vi "uActor_Launch.vi"(6 "Show FP (F)":bool, 8 "error in (no error)":errorcluster, 10 "Actor to Launch":refnum<class "uActor.lvclass">, 11 "Caller Actor in":refnum<class "uActor.lvclass">) -> (0 "error out":errorcluster, 2 "uTransport_uActor":refnum<class "uTransport_uActor.lvclass">, 3 "Caller Actor out":refnum<class "uActor.lvclass">)   [LabVIEW 2021, in "uFramework.lvlib" / "uActor.lvclass"]
doc: "Launch a new Actor. This will be a root actor if no caller actors are wired in."
uses:
  uActor.lvclass
  uTransport_uActor/uTransport_uActor.lvclass
  uTransport_uActor/uTransport_uActor.lvclass/uTransport_uActor.ctl
  uActor.lvclass/uActor.ctl
  uActor.vi
  uMsg/uMsg.lvclass
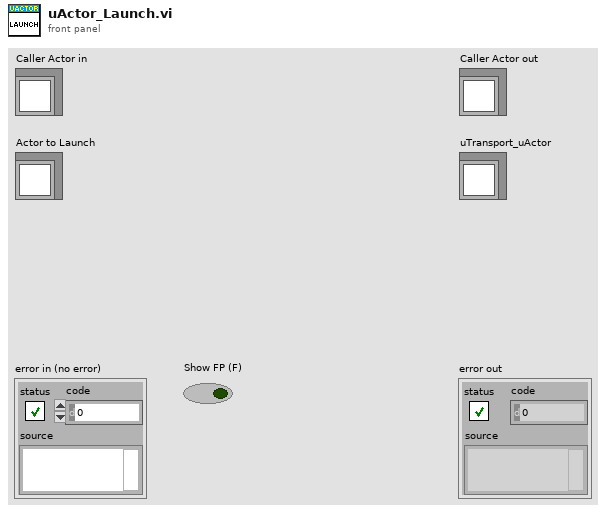
[diagram p1: front panel]
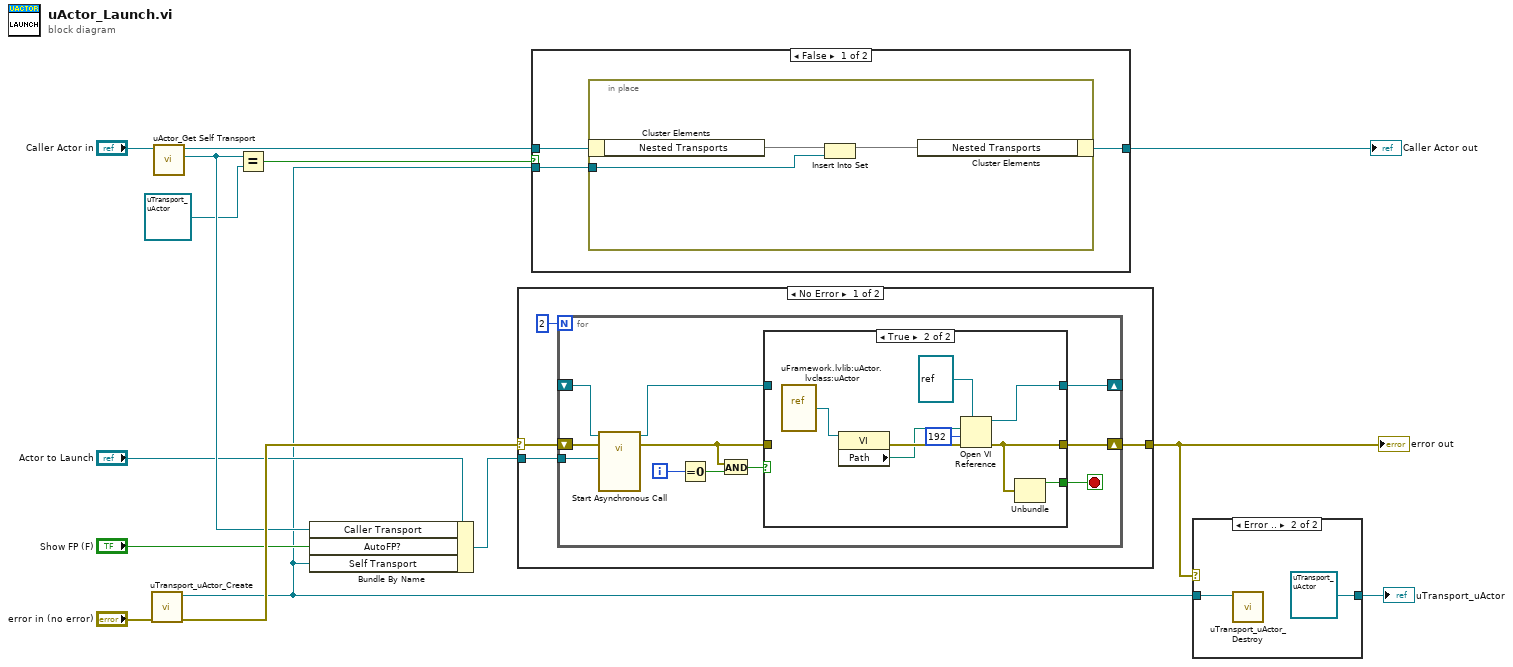
[diagram p0: block diagram]
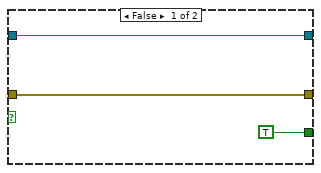
[diagram p2: hidden frame]
diagram:
  n1 = call "uTransport_uActor_Create.vi"("error in (no error)"="error in (no error)") -> ("error out"=w14:errorcluster, "uTransport_uActor out"=w2:refnum<class "uTransport_uActor.lvclass">)  [unwired: 9 in]
  n2 = call "uActor_Get Self Transport.vi"("uActor in"="Caller Actor in") -> ("Actor Transport"=w9:refnum<class "uTransport_uActor.lvclass">, "uActor out"=w7:refnum<class "uActor.lvclass">)  [unwired: 9 in]
  n3 = Equal?(x=w9, y=refnum<class "uTransport_uActor.lvclass"> refnum ("uFramework.lvlib:uTransport_uActor.lvclass")) -> (x = y?=w8:bool)
  n4 = Bundle By Name(cluster="Actor to Launch", "Caller Transport"=w9, "AutoFP?"="Show FP (F)", "Self Transport"=w2) -> (w13:refnum<class "uActor.lvclass">)
  n5 = case shown="No Error" w14 {
    selector: w14 -> [w15 w41]
    tunnel: w13 -> [w18 _]
    tunnel: [w17 w41] -> w5
    frame No Error {
      n6 = for {
        N: 2 -> [_]
        tunnel: w18 -> [w29]
        shift-right: [w25] -> w17
        shift-left: w15 -> [w28]
        shift-right: [w26] -> _
        shift-left: _ -> [w27]
        i -> [w24]
        stop <- w19 stop-if-true
        n7 = call-by-ref "Start Asynchronous Call"(reference=w27, error in=w28, "uActor in"=w29) -> (reference out=w23:refnum<vi>, error out=w20:errorcluster)  [unwired: 9 in, 2 out]
        n8 = Equal To 0?(x=w24) -> (x = 0?=w21:bool)
        n9 = And(x=w20, y=w21) -> (x .and. y?=w22:bool)
        n10 = case shown="True" w22 {
          tunnel: w20 -> [w31 _]
          tunnel: [w32 w35] -> w26
          tunnel: [w31 w34] -> w25
          tunnel: w23 -> [w32 _]
          tunnel: [TRUE w33] -> w19
          frame False {
          }
          frame True {
            n11 = vi-ref "uFramework.lvlib:uActor.lvclass:uActor.vi"() -> (w37:refnum<vi>)
            n12 = property class="VI"(reference=w37) -> (error out=w40:errorcluster, "Path"=w39:path)  [unwired: 1 in, 1 out]
            n13 = Open VI Reference(type specifier VI Refnum (for type only)=refnum<vi> refnum, vi path=w39, options=192, error in (no error)=w40) -> (vi reference=w35:refnum<vi>, error out=w34:errorcluster)  [unwired: 2 in]
            n14 = Unbundle(w34) -> ("status"=w33:bool)  [unwired: 2 out]
          }
        }
      }
    }
    frame Error {
    }
  }
  "error out" <- w5
  n15 = case shown="False" w8 {
    tunnel: w7 -> [w44 w48]
    tunnel: [w42 w48] -> w6
    tunnel: w2 -> [w43 _]
    frame False {
      n16 = in-place {
        in-place-border: w43 -> [w45]
        n17 = in-place-cluster #1(w44) -> ("Nested Transports"=w46:set{refnum<class "uTransport_uActor.lvclass">})
        n18 = Insert Into Set(10:w45, 11:w46) -> (3:w47:set{refnum<class "uTransport_uActor.lvclass">})  [unwired: 1 out]
        n19 = in-place-cluster #1("Nested Transports"=w47) -> (w42:refnum<class "uActor.lvclass">)
      }
    }
    frame True {
      # "Attempting to launch a root actor. No caller provided."
    }
  }
  "Caller Actor out" <- w6
  n20 = case shown="Error .." w5 {
    tunnel: w2 -> [w49 w51]
    tunnel: [w49 refnum<class "uTransport_uActor.lvclass"> refnum] -> w12
    frame No Error {
    }
    frame Error {
      n21 = call "uTransport_uActor_Destroy.vi"("uTransport_uActor in"=w51) -> ()  [unwired: 9 in, 2 out]
    }
  }
  "uTransport_uActor" <- w12
